vi "sub_DL950_result-parsing.vi"   [LabVIEW 2019]
uses:
  _ctrl/rw.ctl
types:
  T1 = typedef "rw.ctl" = enum16{"read", "write"}
  T2 = typedef "DL950_wfms.ctl" = cluster{"wfms":waveform(dbl)[], "Waveform_2":cluster{"t0":dbl, "dt":dbl, "Y":dbl[][]}, "items":dbl[][], "da950_array":dbl[]}
  T3 = typedef "measure_rc.ctl" = cluster{"입력카운트":dbl, "출력카운트":dbl, "충전전압 98 V":dbl, "충전전압 98 초":dbl, "충전전압 63V":dbl, "충전전압 63초":dbl, "충전전류 37A":dbl, "충전전류 37초":dbl, "입력전압":dbl, "방전전압":dbl, "온도":dbl, "전압강하":dbl, "입력전류 RMS":dbl, "출력전압 + 평균 63%":dbl, "출력전류 RMS":dbl, "접촉저항":dbl, "Rising Time 63%":dbl, "Rising Time 98%":dbl, "Failing Time 37%":dbl, "출력전압 - 평균 63%":dbl, "접촉저항":dbl, "출력전류 평균 63%":dbl, "tbd2":dbl, "tbd3":dbl, "tbd5":dbl, "tbd6":dbl, "tbd7":dbl, "tbd8":dbl, "tbd9":dbl, "tbd4":dbl}
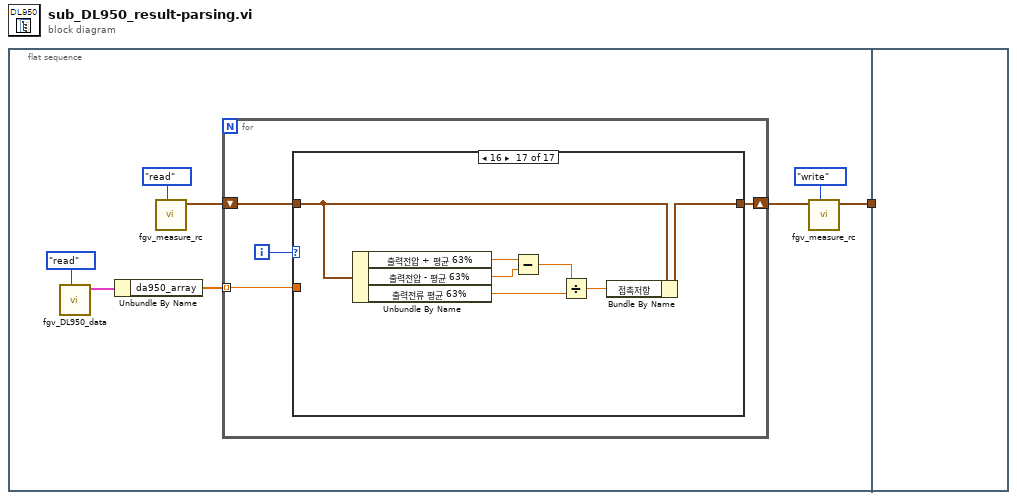
[diagram p0: block diagram]
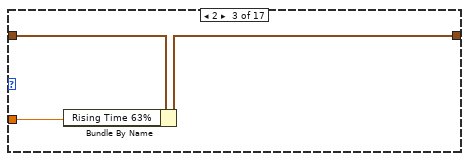
[diagram p4: hidden frame]
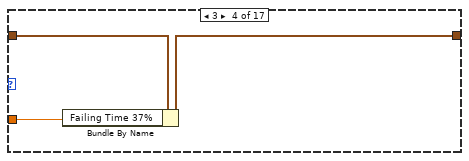
[diagram p5: hidden frame]
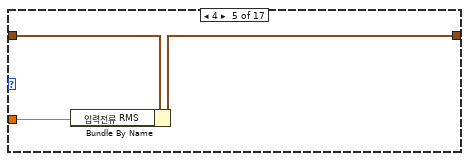
[diagram p6: hidden frame]
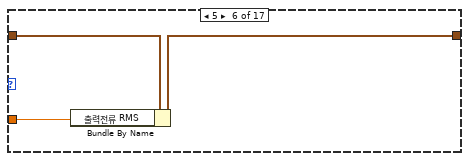
[diagram p7: hidden frame]
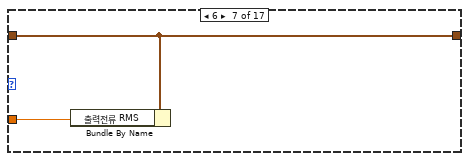
[diagram p8: hidden frame]
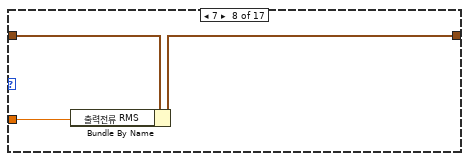
[diagram p9: hidden frame]
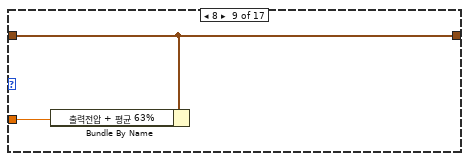
[diagram p10: hidden frame]
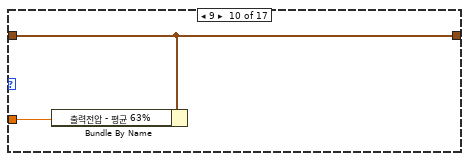
[diagram p11: hidden frame]
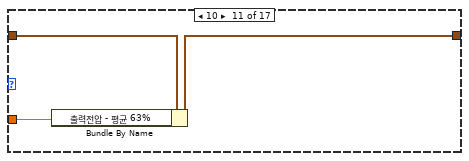
[diagram p12: hidden frame]
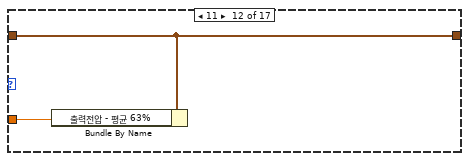
[diagram p13: hidden frame]
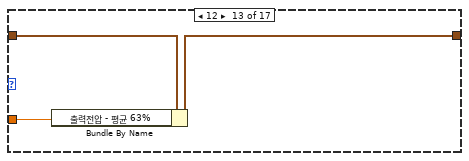
[diagram p14: hidden frame]
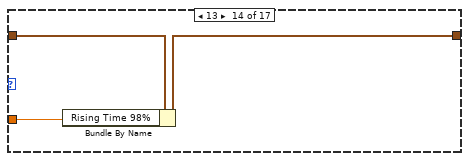
[diagram p15: hidden frame]
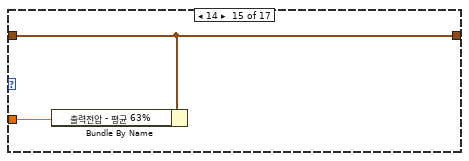
[diagram p16: hidden frame]
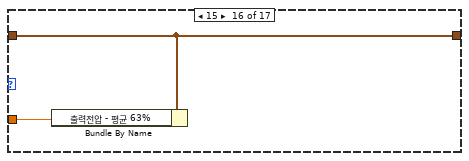
[diagram p17: hidden frame]
diagram:
  n1 = flat-sequence {
    tunnel: [w2] -> w1
    tunnel: w1 -> [_]
    frame #0 {
      n2 = call "fgv_DL950_data.vi"("cmd"=rw."read") -> ("DL950 wfm 2"=w6:T2)  [unwired: 9 in, 1 out]
      n3 = Unbundle By Name(w6) -> ("da950_array"=w5:dbl[])
      n4 = call "fgv_measure_rc.vi"("cmd"=rw."read") -> ("measure_rc 2"=w4:T3)  [unwired: 10 in]
      n5 = for {
        tunnel: w5 -> [w10] mode=indexing
        shift-right: [w11] -> w3
        shift-left: w4 -> [w12]
        i -> [w13]
        n6 = case shown="16" w13 {
          tunnel: w12 -> [w14 w15 w18 w21 w24 w27 w28 w31 w33 w35 w38 w40 w43 w46 w48 w50 w57]
          tunnel: [w14 w15 w17 w20 w23 w26 w28 w30 w33 w35 w37 w40 w42 w45 w48 w50 w58] -> w11
          tunnel: w10 -> [_ _ w16 w19 w22 w25 w29 w32 w34 w36 w39 w41 w44 w47 w49 w51 _]
          frame 0, Default {
          }
          frame 1 {
          }
          frame 2 {
            n7 = Bundle By Name(cluster=w18, "Rising Time 63%"=w16) -> (w17:T3)
          }
          frame 3 {
            n8 = Bundle By Name(cluster=w21, "Failing Time 37%"=w19) -> (w20:T3)
          }
          frame 4 {
            n9 = Bundle By Name(cluster=w24, "입력전류 RMS"=w22) -> (w23:T3)
          }
          frame 5 {
            n10 = Bundle By Name(cluster=w27, "출력전류 RMS"=w25) -> (w26:T3)
          }
          frame 6 {
            n11 = Bundle By Name(cluster=w28, "출력전류 RMS"=w29) -> ()  [unwired: 1 out]
          }
          frame 7 {
            n12 = Bundle By Name(cluster=w31, "출력전류 RMS"=w32) -> (w30:T3)
          }
          frame 8 {
            n13 = Bundle By Name(cluster=w33, "출력전압 + 평균 63%"=w34) -> ()  [unwired: 1 out]
          }
          frame 9 {
            n14 = Bundle By Name(cluster=w35, "출력전압 - 평균 63%"=w36) -> ()  [unwired: 1 out]
          }
          frame 10 {
            n15 = Bundle By Name(cluster=w38, "출력전압 - 평균 63%"=w39) -> (w37:T3)
          }
          frame 11 {
            n16 = Bundle By Name(cluster=w40, "출력전압 - 평균 63%"=w41) -> ()  [unwired: 1 out]
          }
          frame 12 {
            n17 = Bundle By Name(cluster=w43, "출력전압 - 평균 63%"=w44) -> (w42:T3)
          }
          frame 13 {
            n18 = Bundle By Name(cluster=w46, "Rising Time 98%"=w47) -> (w45:T3)
          }
          frame 14 {
            n19 = Bundle By Name(cluster=w48, "출력전압 - 평균 63%"=w49) -> ()  [unwired: 1 out]
          }
          frame 15 {
            n20 = Bundle By Name(cluster=w50, "출력전압 - 평균 63%"=w51) -> ()  [unwired: 1 out]
          }
          frame 16 {
            n21 = Unbundle By Name(w57) -> ("출력전압 + 평균 63%"=w56:dbl, "출력전압 - 평균 63%"=w55:dbl, "출력전류 평균 63%"=w53:dbl)
            n22 = Subtract(x=w56, y=w55) -> (x-y=w54:dbl)
            n23 = Divide(x=w54, y=w53) -> (x/y=w52:dbl)
            n24 = Bundle By Name(cluster=w57, "접촉저항"=w52) -> (w58:T3)
          }
        }
      }
      n25 = call "fgv_measure_rc.vi"("cmd"=rw."write", "measure_rc"=w3) -> ("measure_rc 2"=w2:T3)  [unwired: 9 in]
    }
    frame #1 {
    }
  }
